vi "[SubV]IEncoder_PosVel.vi"(2 "SPI Reference In in":T1 {"SPI Configuration"."Frame Length" min=1 max=16}) -> (0 "ENC1_Position":dbl, 1 "ENC2_Position":dbl, 3 "ENC1_Velocity":dbl, 4 "ENC2_Velocity":dbl, 7 "SPI Reference In out":T1 {"SPI Configuration"."Frame Length" min=1 max=16})   [LabVIEW 2017]
uses:
  <vilib>/myRIO/Instrument Drivers/Onboard IO/SPI/SPI.lvlib
  <vilib>/myRIO/Express VI/Onboard IO/DO/DO Express VI.xnode
  <vilib>/myRIO/Instrument Drivers/Onboard IO/DIO/vis/Write.vi
  <vilib>/myRIO/Instrument Drivers/Onboard IO/DIO/DIO.lvlib
  <vilib>/myRIO/Common/Instrument Driver Framework/myRIO v1.0/DIO/typedefs/DIO Channels Enum.ctl
  <vilib>/myRIO/Common/Instrument Driver Framework/myRIO v1.0/DIO/typedefs/DIO Channels List.ctl
  <vilib>/myRIO/Common/Instrument Driver Framework/Utilities/typedefs/Generic FPGA Reference.ctl
  <vilib>/myRIO/Common/Instrument Driver Framework/Utilities/typedefs/myRIO v1.0 Reference.ctl
  <vilib>/myRIO/Common/Instrument Driver Framework/Utilities/typedefs/Hardware Version Enum.ctl
  <vilib>/myRIO/Common/Instrument Driver Framework/Utilities/typedefs/myRIO Generic Hardware Reference.ctl
  <vilib>/myRIO/Instrument Drivers/Onboard IO/DIO/typedefs/DIO Reference.ctl
  <vilib>/myRIO/Instrument Drivers/Onboard IO/DIO/vis/myRIO DIO Open.xnode
  <vilib>/myRIO/Common/Instrument Driver Framework/Utilities/vis/Is FPGA Ref Available.vi
  <vilib>/myRIO/Common/Instrument Driver Framework/myRIO v1.0/DIO/vis/myRIO v1.1 Open DIO.vi
  <vilib>/userdefined/High Color/nirio_resource_hc.ctl
  <vilib>/myRIO/Common/Instrument Driver Framework/myRIO v1.0/SPI/typedefs/SPI Channels Enum.ctl
  <vilib>/myRIO/Common/Instrument Driver Framework/myRIO v1.0/SPI/typedefs/SPI Clock Phase.ctl
  <vilib>/myRIO/Common/Instrument Driver Framework/myRIO v1.0/SPI/typedefs/SPI Clock Polarity.ctl
  <vilib>/myRIO/Common/Instrument Driver Framework/myRIO v1.0/SPI/typedefs/SPI Data Direction.ctl
  <vilib>/myRIO/Common/Instrument Driver Framework/myRIO v1.0/SPI/typedefs/SPI Frame Length.ctl
  <vilib>/myRIO/Instrument Drivers/Onboard IO/SPI/typedefs/SPI Configuration.ctl
  <vilib>/myRIO/Instrument Drivers/Onboard IO/SPI/typedefs/SPI Reference.ctl
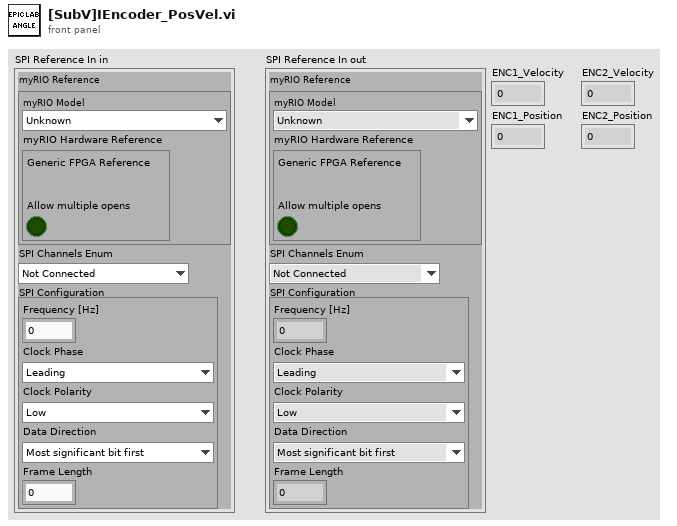
[diagram p1: front panel]
types:
  T1 = typedef "SPI.lvlib/SPI Reference.ctl" = cluster{"myRIO Reference":T2, "SPI Channels Enum":T6, "SPI Configuration":T7}
  T2 = typedef "myRIO Generic Hardware Reference.ctl" = cluster{"myRIO Model":T3, "myRIO Hardware Reference":T4}
  T3 = typedef "Hardware Version Enum.ctl" = enum16{"Unknown", "myRIO-1900", "myRIO-1950", "roboRIO", "NI ELVIS RIO CM"}
  T4 = typedef "myRIO v1.0 Reference.ctl" = cluster{"Generic FPGA Reference":T5, "Allow multiple opens":bool}
  T5 = typedef "Generic FPGA Reference.ctl" = refnum<k20>
  T6 = typedef "SPI Channels Enum.ctl" = enum16{"Not Connected", "A/SPI", "B/SPI", "SPI/SPI"}
  T7 = typedef "SPI.lvlib/SPI Configuration.ctl" = cluster{"Frequency [Hz]":dbl, "Clock Phase":T8, "Clock Polarity":T9, "Data Direction":T10, "Frame Length":T11}
  T8 = typedef "SPI Clock Phase.ctl" = enum8{"Leading", "Trailing"}
  T9 = typedef "SPI Clock Polarity.ctl" = enum8{"Low", "High"}
  T10 = typedef "SPI Data Direction.ctl" = enum8{"Most significant bit first", "Least significant bit first"}
  T11 = typedef "SPI Frame Length.ctl" = u8
  T12 = typedef "DIO.lvlib/DIO Reference.ctl" = cluster{"myRIO Reference":T2, "DIO Channels List":T13}
  T13 = typedef "DIO Channels List.ctl" = T14[]
  T14 = typedef "DIO Channels Enum.ctl" = enum16{"Not Connected", "C/DIO0", "C/DIO1", "C/DIO2", "C/DIO3", "C/DIO4", "C/DIO5", "C/DIO6", "C/DIO7", "A/DIO0", "A/DIO1", "A/DIO2", "A/DIO3", "A/DIO4", "A/DIO5", "A/DIO6", "A/DIO7", "A/DIO8", "A/DIO9", "A/DIO10", "A/DIO11", "A/DIO12", "A/DIO13", "A/DIO14", "A/DIO15", "B/DIO0", "B/DIO1", "B/DIO2", "B/DIO3", "B/DIO4", "B/DIO5", "B/DIO6", "B/DIO7", "B/DIO8", "B/DIO9", "B/DIO10", "B/DIO11", "B/DIO12", "B/DIO13", "B/DIO14", "B/DIO15", "LED0", "LED1", "LED2", "LED3", "Button0", "DIO/DIO0", "DIO/DIO1", "DIO/DIO2", "DIO/DIO3", "DIO/DIO4", "DIO/DIO5", "DIO/DIO6", "DIO/DIO7", "DIO/DIO8", "DIO/DIO9", "SPI/CS0", "SPI/CS1", "SPI/CS2", "SPI/CS3", "LED RADIO (Green)", "LED RADIO (Red)", "LED COMM (Green)", "LED COMM (Red)", "LED MODE (Green)", "LED MODE (Red)"}
  T15 = typedef "nirio_resource_hc.ctl" = tag
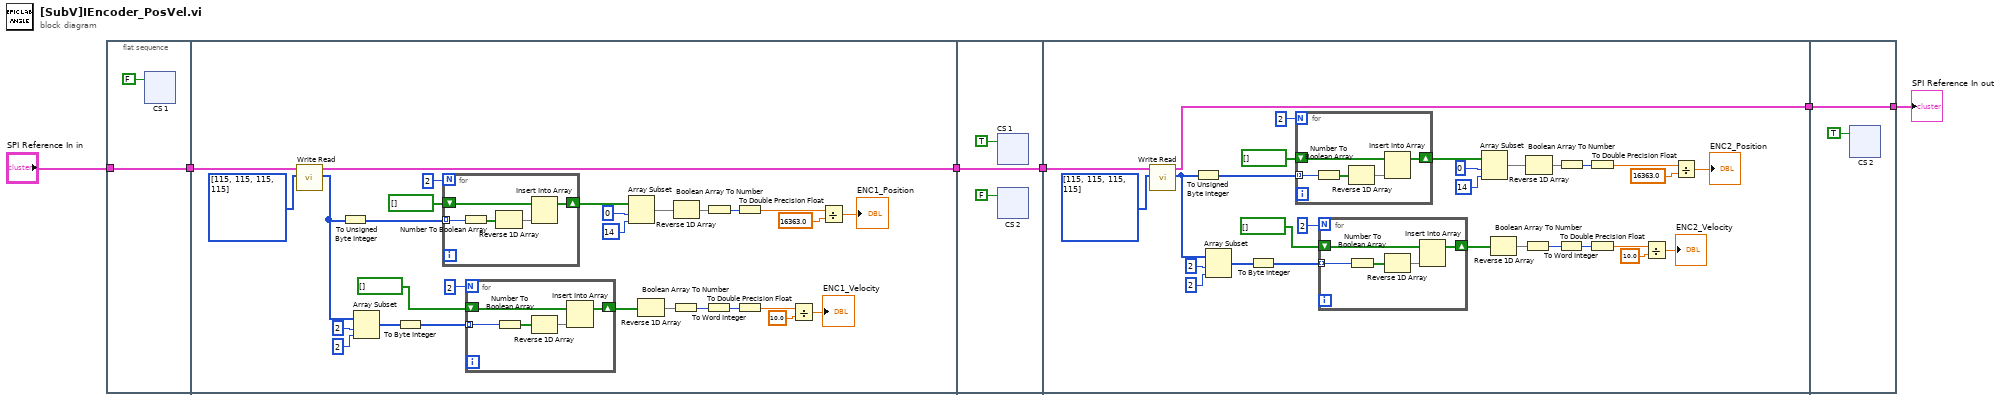
[diagram p0: block diagram]
diagram:
  n1 = flat-sequence {
    tunnel: [w8] -> w5
    tunnel: "SPI Reference In in" -> [w8]
    tunnel: w5 -> [w57]
    tunnel: [w56] -> w4
    tunnel: w4 -> [w85]
    tunnel: [w85] -> w3
    tunnel: w3 -> [w158]
    tunnel: [w157] -> w2
    tunnel: w2 -> [w196]
    tunnel: [w196] -> w1
    frame #0 {
      n2 = xnode "CS 1"("A/DIO1 (Pin 13)"=FALSE) -> ()  [unwired: 1 in, 1 out]
    }
    frame #1 {
      n3 = call <vilib>:"Write Read.vi"("Frames to Write"=u16[] [115, 115, 115, 115], "SPI Ref In"=w57) -> ("Frames Read"=w63:u16[], "SPI Ref Out"=w56:T1)  [unwired: 7 in, 1 out]
      n4 = To Unsigned Byte Integer(number=w63) -> (unsigned 8bit integer=w72:u8[])
      n5 = Array Subset(array=w63, index=2, length=2) -> (w60:u16[])
      n6 = To Byte Integer(number=w60) -> (8bit integer=w54:i8[])
      n7 = for {
        N: 2 -> [_]
        tunnel: w72 -> [w82] mode=indexing
        shift-right: [w80] -> w65
        shift-left: bool[] [] -> [w81]
        n8 = Number To Boolean Array(number=w82) -> (Boolean array=w79:bool[])
        n9 = Reverse 1D Array(array=w79) -> (reversed array=w78:bool[])
        n10 = Insert Into Array(array=w81, new element=w78) -> (w80:bool[])  [unwired: 1 in]
      }
      n11 = for {
        N: 2 -> [_]
        tunnel: w54 -> [w74] mode=indexing
        shift-right: [w75] -> w55
        shift-left: bool[] [] -> [w73]
        n12 = Number To Boolean Array(number=w74) -> (Boolean array=w77:bool[])
        n13 = Reverse 1D Array(array=w77) -> (reversed array=w76:bool[])
        n14 = Insert Into Array(array=w73, new element=w76) -> (w75:bool[])  [unwired: 1 in]
      }
      n15 = Array Subset(array=w65, index=0, length=14) -> (w66:bool[])
      n16 = Reverse 1D Array(array=w55) -> (reversed array=w64:bool[])
      n17 = Boolean Array To Number(Boolean array=w64) -> (number=w59:u16)
      n18 = Reverse 1D Array(array=w66) -> (reversed array=w67:bool[])
      n19 = To Word Integer(number=w59) -> (16bit integer=w51:i16)
      n20 = Boolean Array To Number(Boolean array=w67) -> (number=w49:u16)
      n21 = To Double Precision Float(number=w49) -> (double precision float=w48:dbl)
      n22 = To Double Precision Float(number=w51) -> (double precision float=w52:dbl)
      n23 = Divide(x=w52, y=10.0) -> (x/y=→"ENC1_Velocity":dbl)
      n24 = Divide(x=w48, y=16363.0) -> (x/y=→"ENC1_Position":dbl)
    }
    frame #2 {
      n25 = xnode "CS 1"("A/DIO1 (Pin 13)"=TRUE) -> ()  [unwired: 1 in, 1 out]
      n26 = xnode "CS 2"("A/DIO2 (Pin 15)"=FALSE ("A/DIO1 (Pin 13)")) -> ()  [unwired: 1 in, 1 out]
    }
    frame #3 {
      n27 = call <vilib>:"Write Read.vi"("Frames to Write"=u16[] [115, 115, 115, 115], "SPI Ref In"=w158) -> ("Frames Read"=w175:u16[], "SPI Ref Out"=w157:T1)  [unwired: 7 in, 1 out]
      n28 = To Unsigned Byte Integer(number=w175) -> (unsigned 8bit integer=w184:u8[])
      n29 = Array Subset(array=w175, index=2, length=2) -> (w172:u16[])
      n30 = To Byte Integer(number=w172) -> (8bit integer=w168:i8[])
      n31 = for {
        N: 2 -> [_]
        tunnel: w184 -> [w194] mode=indexing
        shift-right: [w192] -> w177
        shift-left: bool[] [] -> [w193]
        n32 = Number To Boolean Array(number=w194) -> (Boolean array=w191:bool[])
        n33 = Reverse 1D Array(array=w191) -> (reversed array=w190:bool[])
        n34 = Insert Into Array(array=w193, new element=w190) -> (w192:bool[])  [unwired: 1 in]
      }
      n35 = for {
        N: 2 -> [_]
        tunnel: w168 -> [w186] mode=indexing
        shift-right: [w187] -> w169
        shift-left: bool[] [] -> [w185]
        n36 = Number To Boolean Array(number=w186) -> (Boolean array=w189:bool[])
        n37 = Reverse 1D Array(array=w189) -> (reversed array=w188:bool[])
        n38 = Insert Into Array(array=w185, new element=w188) -> (w187:bool[])  [unwired: 1 in]
      }
      n39 = Array Subset(array=w177, index=0, length=14) -> (w178:bool[])
      n40 = Reverse 1D Array(array=w169) -> (reversed array=w176:bool[])
      n41 = Boolean Array To Number(Boolean array=w176) -> (number=w171:u16)
      n42 = Reverse 1D Array(array=w178) -> (reversed array=w179:bool[])
      n43 = To Word Integer(number=w171) -> (16bit integer=w165:i16)
      n44 = Boolean Array To Number(Boolean array=w179) -> (number=w163:u16)
      n45 = To Double Precision Float(number=w163) -> (double precision float=w162:dbl)
      n46 = To Double Precision Float(number=w165) -> (double precision float=w166:dbl)
      n47 = Divide(x=w166, y=10.0) -> (x/y=→"ENC2_Velocity":dbl)
      n48 = Divide(x=w162, y=16363.0) -> (x/y=→"ENC2_Position":dbl)
    }
    frame #4 {
      n49 = xnode "CS 2"("A/DIO2 (Pin 15)"=TRUE ("A/DIO1 (Pin 13)")) -> ()  [unwired: 1 in, 1 out]
    }
  }
  "SPI Reference In out" <- w1
